vi "Configurar.vi"(8 "error in (no error)":errorcluster, 11 "Simulada in":refnum<class "Simulada.lvclass">) -> (0 "error out":errorcluster, 3 "Simulada out":refnum<class "Simulada.lvclass">)   [LabVIEW 2020, in "Simulada.lvclass"]
uses:
  Simulada.lvclass
  Simulada.lvclass/Simulada.ctl
  Write RutaImagenes.vi
  Abstracta/Camara/Camara.lvclass
panel:
  in  "Apply":bool
  in  "Path":path
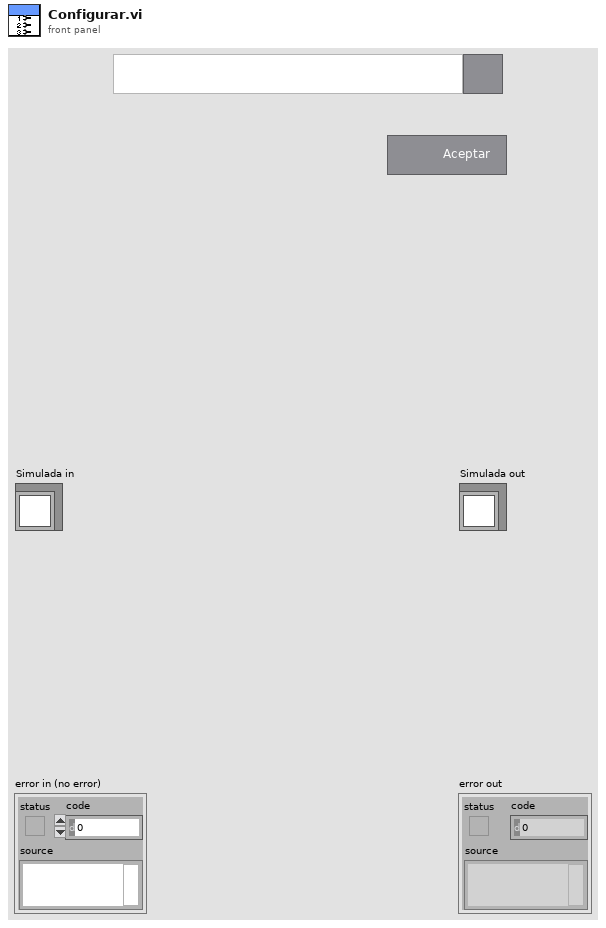
[diagram p1: front panel]
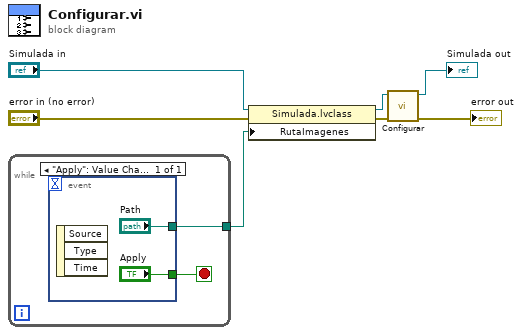
[diagram p0: block diagram]
diagram:
  n1 = while {
    tunnel: [w8] -> w5
    stop <- w9 stop-if-true
    n2 = event shown="[0] \"Apply\": Value Change" {
      selector: _ -> [_]
      dyn-events: _ -> [_]
      timeout: _ -> [_]
      tunnel: ["Apply"] -> w9
      tunnel: ["Path"] -> w8
      event "Apply": Value Change {
        n3 = event-data() -> ()  [unwired: 1 in, 3 out]
      }
    }
  }
  n4 = property class="Simulada.lvclass"(reference="Simulada in", error in="error in (no error)", "RutaImagenes"=w5) -> (reference out=w4:refnum<class "Simulada.lvclass">, error out=w2:errorcluster)
  n5 = call-parent "Configurar.vi"("error in (no error)"=w2, "Camara in"=w4) -> ("error out"=→"error out":errorcluster, "Camara out"=→"Simulada out":refnum<class "Simulada.lvclass">)  [unwired: 8 in]
